vi "Register Logger.vi"(4 "dialog on failure? (T)":bool=TRUE, 5 "minimum log level (Info)":T1=enum."Info", 6 "enabled? (T)":bool=TRUE, 7 "name (\"Default\")":string="Default", 8 "error in (no error)":errorcluster, 9 "log handler (file handler)":refnum<class "Formatting Handler.lvclass">, 10 "log filter (none)":refnum<class "Filter.lvclass">, 11 "logger scope (all)":refnum<class "Scope.lvclass">) -> (0 "error out":errorcluster)   [LabVIEW 2018, in "Logging.lvlib"]
uses:
  Logging.lvlib
  Log Levels.ctl
  extension/formatting_handler_interface/Formatting Handler.lvclass
  extension/filter_interface/Filter.lvclass
  extension/scope_interface/Scope.lvclass
  logger_class/Logger.lvclass
  registry/Registry.lvlib
panel:
  # "Connector Pane"
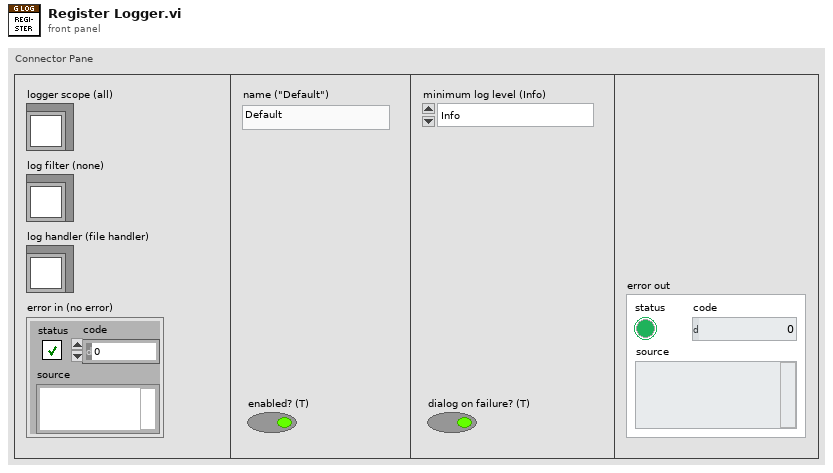
[diagram p1: front panel]
types:
  T1 = typedef "Logging.lvlib/Log Levels.ctl" = enum16{"Trace", "Debug", "Info", "Warning", "Error", "Critical"}
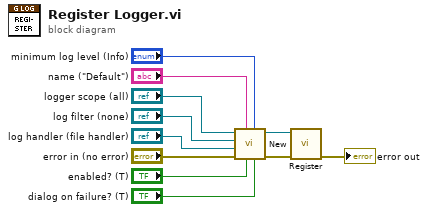
[diagram p0: block diagram]
diagram:
  n1 = call "New.vi"("dialog on failure? (T)"="dialog on failure? (T)", "minimum log level (Info)"="minimum log level (Info)", "enabled? (T)"="enabled? (T)", "name (\"Default\")"="name (\"Default\")", "error in (no error)"="error in (no error)", "log handler (file handler)"="log handler (file handler)", "log filter (none)"="log filter (none)", "logger scope (all)"="logger scope (all)") -> ("error out"=w10:errorcluster, "logger"=w11:refnum<class "Logger.lvclass">)  [unwired: 2 in]
  n2 = call "Register.vi"("error in (no error)"=w10, "logger in"=w11) -> ("error out"=→"error out":errorcluster)  [unwired: 9 in]
